vi "scaler_analog_digital_2channels_example.vi"() -> ()   [LabVIEW 2018]
uses:
  <vilib>/Platform/TimedLoop/XDataNode/timing_clust.ctl
  <vilib>/Platform/TimedLoop/XDataNode/nitl_modes.ctl
  <vilib>/Platform/TimedLoop/XDataNode/wakeup.ctl
  <vilib>/rvi/Emulation/niFpgaGetClockAttributes.vi
  <vilib>/rvi/Emulation/niFpgaSctlEmulationGetInTimedLoop.vi
  <vilib>/rvi/Emulation/niFpgaEmulationReportErrorSimple.vi
  <vilib>/rvi/eio/common/nirviEmuTemplateMethod_errors.vi
  <vilib>/rvi/Emulation/niFpgaProcessEmulError.vi
  <vilib>/rvi/Emulation/niFpgaCriticalErrorInLSC.vi
  <vilib>/eio/EIONode/EIONode.xnode
  <vilib>/Platform/TimedLoop/XDataNode/XDataNode.xnode
  <vilib>/Platform/TimedLoop/XDataNode/XDNodeRunTimeDep.lvlib
  lib/Scaler-EPICS/scaler.lvlib
panel:
  out "Looptime":u32
  in  "AnalogInputs_Scaler_Analog":u32[](array[numeric])=[0, 0]
  in  "PresetValues_Scaler_Analog":u32[](array[numeric])=[0, 0]
  in  "Gate_Scaler_Analog":bool[](array[boolean])=[FALSE, FALSE]
  in  "OneShot_Scaler_Analog":bool
  in  "Enable_Scaler_Analog":bool
  out "Counter_Scaler_Analog":u32[](array[numeric])
  out "Done_Scaler_Analog":bool
  in  "sample_Scaler_Analog":bool
  in  "OneShot_Scaler_Digital":bool
  in  "Enable_Scaler_Digital":bool
  in  "Gate_Scaler_Digital":bool[](array[boolean])=[FALSE, FALSE]
  out "Done_Scaler_Digital":bool
  out "Counter_Scaler_Digital":u32[](array[numeric])
  in  "PresetValues_Scaler_Digital":u32[](array[numeric])=[0, 0]
  in  "Pulse_Scaler_Digital":bool[](array[boolean])=[FALSE]
  # "** Pay attention to the single cycle timed loop clock speed. **"
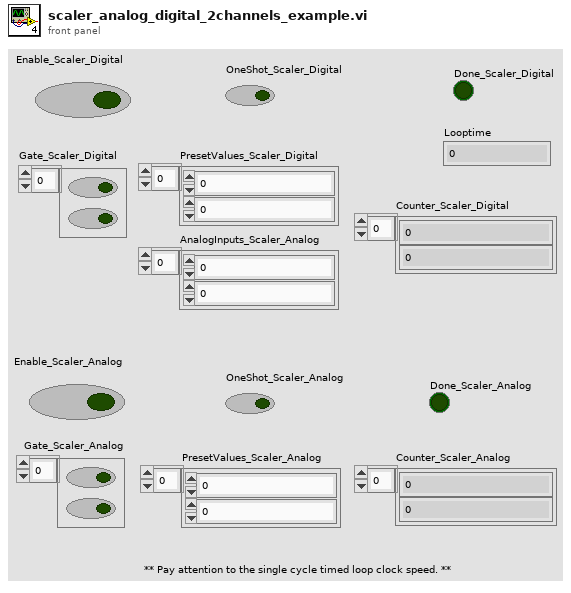
[diagram p1: front panel]
types:
  T1 = typedef "XDNodeRunTimeDep.lvlib/timing_clust.ctl" = cluster{"Expected End [f-1]":u64, "Actual End [f-1]":u64, "Finished Late? [f-1]":bool, "Expected End [i-1]":u64, "Actual End [i-1]":u64, "Finished Late? [i-1]":bool, "Expected Start [i]":u64, "Actual Start [i]":u64, "Expected Start [f]":u64, "Actual Start [f]":u64, "Source Name":string, "Structure Name":string, "Period":i64, "Deadline":i64, "Offset":i64, "Start":i64, "Priority":i32, "Timeout":i32, "Mode":T2, "Wakeup Reason":T3, "Error":errorcluster, "Source Type":string, "Secondary Source Type":string, "Global End Time":u64, "Global Start Time":u64, "Frame Duration":u64, "Iteration Duration":u64, "Assigned CPU":i32, "I/O Scan Engine Mode":u32}
  T2 = typedef "XDNodeRunTimeDep.lvlib/nitl_modes.ctl" = enum32{"No Change", "Process missed periods, maintain original phase", "Discard missed periods, maintain original phase", "Process missed periods, ignore original phase", "Discard missed periods, ignore original phase"}
  T3 = typedef "XDNodeRunTimeDep.lvlib/wakeup.ctl" = enum32{"Normal", "Aborted", "Asynchronous wakeup", "Timing source error", "Timed loop error", "Timeout"}
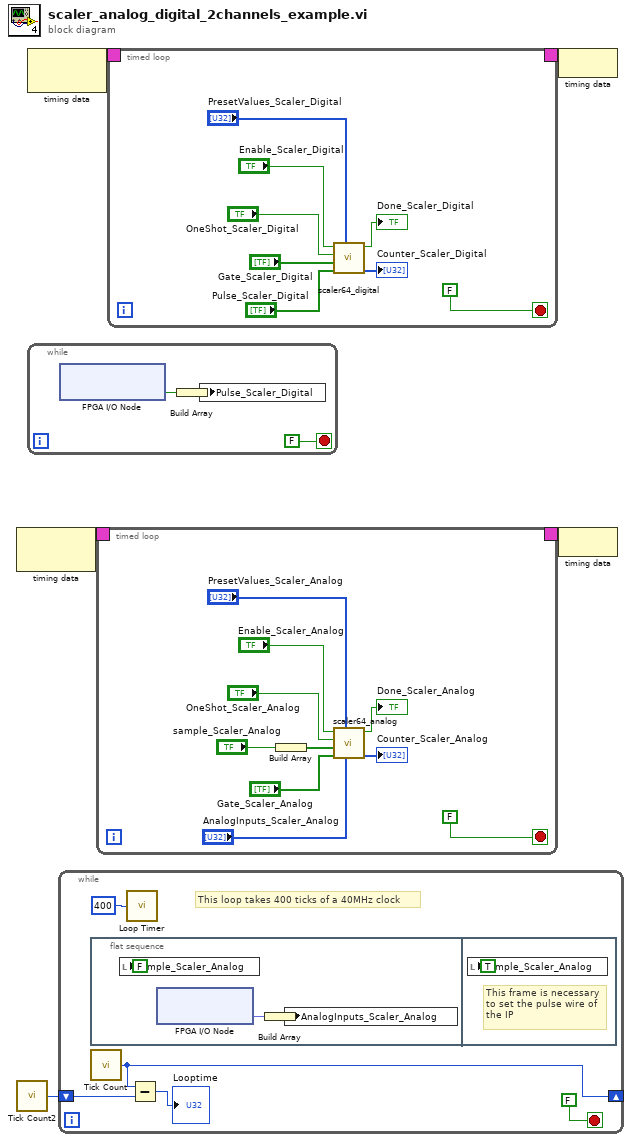
[diagram p0: block diagram]
diagram:
  n1 = node-c288() -> (w3:T1)  [unwired: 1 in]
  n2 = call "Tick Count2"() -> ("Tick Count(Ticks)"=w1:u32)
  n3 = node-c288() -> (w5:T1)  [unwired: 1 in]
  n4 = while {
    stop <- FALSE stop-if-true
    n5 = xnode "FPGA I/O Node"() -> ("Mod2/DIO0"=w8:bool)  [unwired: 1 in, 1 out]
    n6 = Build Array(w8) -> (w7:bool[])
    n7 = local write "Pulse_Scaler_Digital"(w7) -> ()
  }
  n8 = while {
    shift-right: [w10] -> _
    shift-left: w1 -> [w11]
    stop <- FALSE stop-if-true
    # "This loop takes 400 ticks of a 40MHz clock"
    n9 = flat-sequence {
      frame #0 {
        n10 = local write "sample_Scaler_Analog"(FALSE) -> ()
        n11 = xnode "FPGA I/O Node"() -> ("Mod4/AI0"=w16:fxp<+/-,20,5>)  [unwired: 1 in, 1 out]
        n12 = Build Array(w16) -> (w15:fxp<+/-,20,5>[])
        n13 = local write "AnalogInputs_Scaler_Analog"(w15) -> ()
      }
      frame #1 {
        # "This frame is necessary to set the pulse wire of the IP"
        n14 = local write "sample_Scaler_Analog"(TRUE ("sample")) -> ()
      }
    }
    n15 = call "Tick Count"() -> ("Tick Count(Ticks)"=w10:u32)
    n16 = call "Loop Timer"("Count(Ticks)"=i16 400) -> ()  [unwired: 1 out]
    n17 = Subtract(x=w10, y=w11) -> (x-y=→"Looptime":u32)
  }
  n18 = timed-loop {
    timing: w3 -> [_]
    timing-out: [_] -> w2
    stop <- FALSE stop-if-true
    n19 = Build Array("sample_Scaler_Analog") -> (w19:bool[])
    n20 = call "scaler64_analog.vi"("AnalogInputs_Scaler"="AnalogInputs_Scaler_Analog", "PresetValues_Scaler"="PresetValues_Scaler_Analog", "Gate_Scaler"="Gate_Scaler_Analog", "Pulse_Scaler"=w19, "OneShot_Scaler"="OneShot_Scaler_Analog", "Enable_Scaler"="Enable_Scaler_Analog") -> ("Counter_Scaler"=→"Counter_Scaler_Analog":u32[], "Done_Scaler"=→"Done_Scaler_Analog":bool)  [unwired: 4 in]
  }
  n21 = timed-loop {
    timing: w5 -> [_]
    timing-out: [_] -> w4
    stop <- FALSE stop-if-true
    n22 = call "scaler64_digital.vi"("PresetValues_Scaler"="PresetValues_Scaler_Digital", "Pulse_Scaler"="Pulse_Scaler_Digital", "Gate_Scaler"="Gate_Scaler_Digital", "OneShot_Scaler"="OneShot_Scaler_Digital", "Enable_Scaler"="Enable_Scaler_Digital") -> ("Counter_Scaler"=→"Counter_Scaler_Digital":u32[], "Done_Scaler"=→"Done_Scaler_Digital":bool)  [unwired: 5 in]
  }
  n23 = node-c288(w4) -> ()
  n24 = node-c288(w2) -> ()
